vi "AskForConnectedSCDs.vi"(7 "DiscoverDevices in":T1, 8 "error in (no error)":errorcluster, 10 "timeout for receiving data [ms]":i32=5000, 11 "Communicator in":refnum<class "Communicator.lvclass">) -> (0 "error out":errorcluster, 1 "SCDs":refnum<class "SCD.lvclass">[](array[class]), 2 "DiscoverDevices out":T1, 3 "Communicator out":refnum<class "Communicator.lvclass">)   [LabVIEW 2020, in "horiba.lvlib" / "DeviceManager.lvlib"]
uses:
  DeviceManager.lvlib
  GenericDevice/GenericDevice.lvclass
  SCD/SCD.lvclass
  Communicator/Communicator.lvclass
  Mono/Monochromator.lvclass
  CCD/CCD.lvclass
  DiscoverDevices (Reply Payload)--cluster.ctl
panel:
  # "Connector Pane"
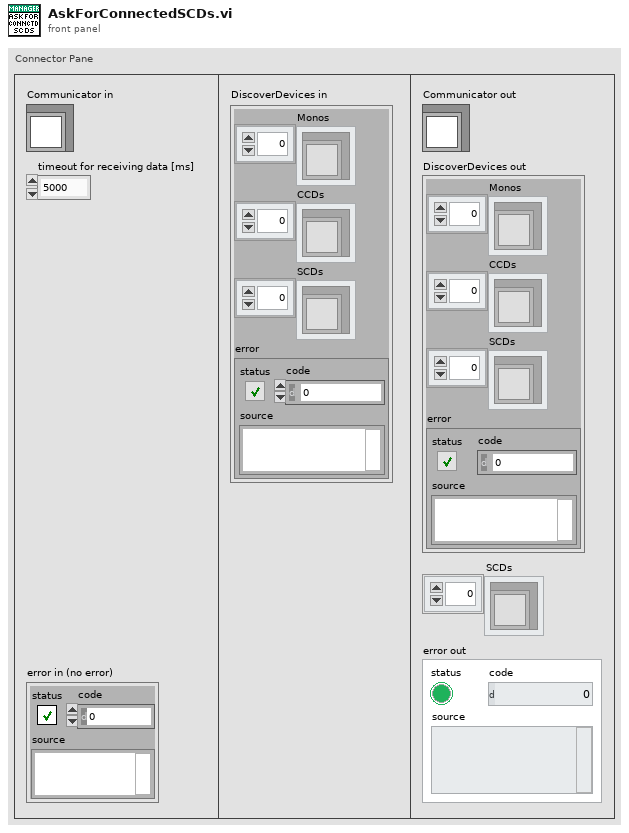
[diagram p1: front panel]
types:
  T1 = typedef "horiba.lvlib/DeviceManager.lvlib/DiscoverDevices (Reply Payload)--cluster.ctl" = cluster{"Monos":refnum<class "Monochromator.lvclass">[], "CCDs":refnum<class "CCD.lvclass">[], "SCDs":refnum<class "SCD.lvclass">[], "error":errorcluster}
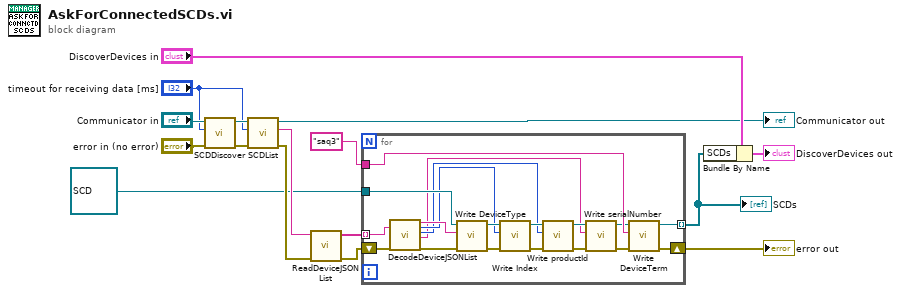
[diagram p0: block diagram]
diagram:
  n1 = call "SCDDiscover.vi"("error in (no error)"="error in (no error)", "Delay between send and receive [ms]"="timeout for receiving data [ms]", "Communicator in"="Communicator in") -> ("error out"=w5:errorcluster, "Communicator out"=w7:refnum<class "Communicator.lvclass">)  [unwired: 5 in, 2 out]
  n2 = call "SCDList.vi"("error in (no error)"=w5, "Delay between send and receive [ms]"="timeout for receiving data [ms]", "Communicator in"=w7) -> ("error out"=w4:errorcluster, "results-JSON"=w10:string, "Communicator out"=→"Communicator out":refnum<class "Communicator.lvclass">)  [unwired: 5 in, 1 out]
  n3 = call "ReadDeviceJSONList.vi"("error in"=w4, "JSON"=w10) -> ("error out"=w12:errorcluster, "table of devices"=w13:string[])  [unwired: 8 in]
  n4 = for {
    tunnel: w13 -> [w32] mode=indexing
    shift-right: [w28] -> w14
    shift-left: w12 -> [w31]
    tunnel: [w29] -> w2 mode=indexing
    tunnel: "saq3" -> [w30]
    tunnel: refnum<class "SCD.lvclass"> refnum ("SCD.lvclass") -> [w21]
    n5 = call "DecodeDeviceJSONList.vi"("JSON"=w32, "error in"=w31) -> ("deviceType"=w20:string, "index"=w19:i32, "productId"=w18:i32, "serialNumber"=w17:string, "error out"=w34:errorcluster)  [unwired: 12 in, 1 out]
    n6 = call-dynamic "Write DeviceType.vi"("error in (no error)"=w34, "device type"=w20, "SCD in"=w21) -> ("error out"=w33:errorcluster, "SCD out"=w35:refnum<class "SCD.lvclass">)  [unwired: 7 in]
    n7 = call-dynamic "Write Index.vi"("error in (no error)"=w33, "Index"=w19, "SCD in"=w35) -> ("error out"=w25:errorcluster, "SCD out"=w27:refnum<class "SCD.lvclass">)  [unwired: 7 in]
    n8 = call-dynamic "Write productId.vi"("error in (no error)"=w25, "productId"=w18, "SCD in"=w27) -> ("error out"=w24:errorcluster, "SCD out"=w26:refnum<class "SCD.lvclass">)  [unwired: 7 in]
    n9 = call-dynamic "Write serialNumber.vi"("error in (no error)"=w24, "serialNumber"=w17, "SCD in"=w26) -> ("error out"=w22:errorcluster, "SCD out"=w23:refnum<class "SCD.lvclass">)  [unwired: 7 in]
    n10 = call-dynamic "Write DeviceTerm.vi"("error in (no error)"=w22, "deviceTerm"=w30, "SCD in"=w23) -> ("error out"=w28:errorcluster, "SCD out"=w29:refnum<class "SCD.lvclass">)  [unwired: 7 in]
  }
  "error out" <- w14
  "SCDs" <- w2
  n11 = Bundle By Name(cluster="DiscoverDevices in", "SCDs"=w2) -> (→"DiscoverDevices out":T1)
